vi "Global 1.vi"() -> ()   [LabVIEW 2012]
panel:
  in  "Table Control":string[][](table)
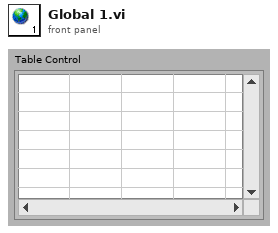
[diagram p1: front panel]
diagram:
